vi "Set Initialization Data - Main UI.vi"(8 "error in":errorcluster, 11 "Host NI 9205 Demo in":refnum<class "Host NI 9205 Demo.lvclass">) -> (0 "error out":errorcluster, 3 "Host NI 9205 Demo out":refnum<class "Host NI 9205 Demo.lvclass">)   [LabVIEW 2017, in "Host NI 9205 Demo.lvclass"]
doc: "In this VI you can set the initialization data of a statically-linked subWorker."
uses:
  Host NI 9205 Demo.lvclass
  Main UI/Initialization Data.ctl
  Main UI/Response Cases.ctl
  <vilib>/addons/_Workers/Library/Case Label.ctl
  Host NI 9205 Demo.lvclass/Host NI 9205 Demo.ctl
  Main UI/Main UI.lvclass
  C:/Program Files (x86)/National Instruments/LabVIEW 2017/vi.lib/addons/_Workers/Library/Classes/Worker/Worker.lvclass
  <vilib>/addons/_Workers/Library/Workers.lvlib
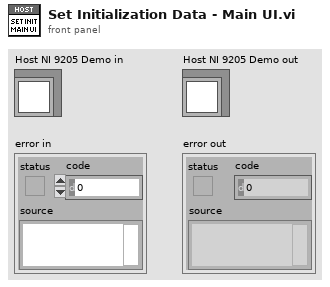
[diagram p1: front panel]
types:
  T1 = typedef "Main UI.lvclass/Initialization Data.ctl" = cluster{"Response Cases":T2}
  T2 = typedef "Main UI.lvclass/Response Cases.ctl" = cluster{"TCP Server Start Listening":T3, "TCP Server Stop Listening":T3, "Start Exiting Application":T3}
  T3 = typedef "Workers.lvlib/Case Label.ctl" = string
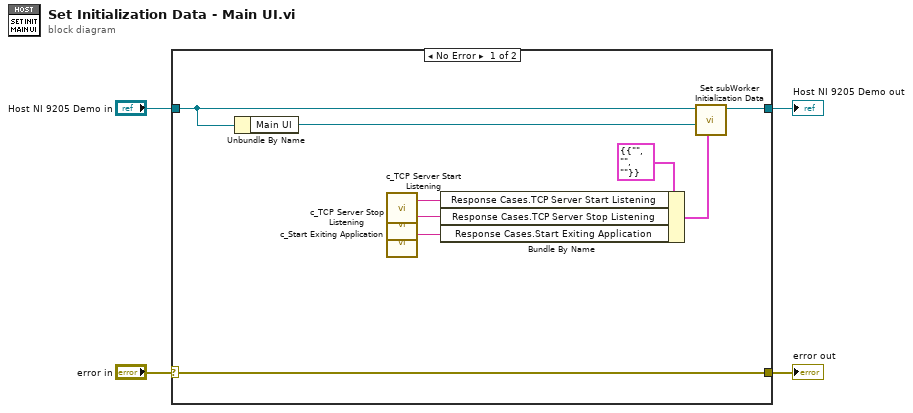
[diagram p0: block diagram]
diagram:
  n1 = case shown="No Error" "error in" {
    selector: "error in" -> [w13 w15]
    tunnel: [w13 w15] -> w3
    tunnel: [w11 w14] -> w2
    tunnel: "Host NI 9205 Demo in" -> [w10 w14]
    frame No Error {
      n2 = Unbundle By Name(w10) -> ("Main UI"=w12:refnum<class "Main UI.lvclass">)
      n3 = call "c_TCP Server Start Listening.vi"() -> ("Case Label"=w7:T3)  [unwired: 1 in]
      n4 = call "c_TCP Server Stop Listening.vi"() -> ("Case Label"=w6:T3)  [unwired: 1 in]
      n5 = call "c_Start Exiting Application.vi"() -> ("Case Label"=w5:T3)  [unwired: 1 in]
      n6 = Bundle By Name(cluster=T1 {"Response Cases"={"TCP Server Start Listening"="", "TCP Server Stop Listening"="", "Start Exiting Application"=""}} ("Initialization Data"), "Response Cases.TCP Server Start Listening"=w7, "Response Cases.TCP Server Stop Listening"=w6, "Response Cases.Start Exiting Application"=w5) -> (w8:T1)
      n7 = call-dynamic "Set subWorker Initialization Data.vi"("Initialization Data"=w8, "subWorker"=w12, "Worker"=w10) -> ("Worker out"=w11:refnum<class "Host NI 9205 Demo.lvclass">)  [unwired: 8 in]
    }
    frame Error {
    }
  }
  "error out" <- w3
  "Host NI 9205 Demo out" <- w2
